vi "Configure Pins.vi"(8 "error in":errorcluster, 11 "2727 in":refnum<class "2727.lvclass">) -> (0 "error out":errorcluster, 3 "2727 out":refnum<class "2727.lvclass">)   [LabVIEW 2019, in "2727.lvlib" / "2727.lvclass"]
uses:
  Library/2727.lvclass
  C:/Users/Public/Documents/Development/builds/Instruments/PRM.lvlibp/Library/PRM.lvclass
  Library/2727.lvclass/2727.ctl
  <instrlib>/ni272xReferenceVIs/ni272xReferenceVIs.llb/ni272x Connector Identifier.ctl
  builds/Instruments/PRM.lvlibp/Accessors/Read NumChans.vi
  <instrlib>/ni272xReferenceVIs/ni272xReferenceVIs.llb/ni272x Connect to Connector 1Chan.vi
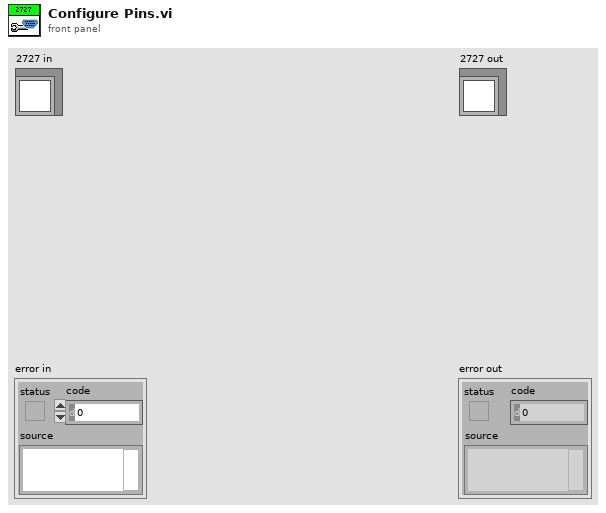
[diagram p1: front panel]
types:
  T1 = typedef "ni272x Connector Identifier.ctl" = enum8{"DUT Connector", "DMM Test Connector"}
  T2 = typedef "ni272x Reference.ctl" = refnum<k20>
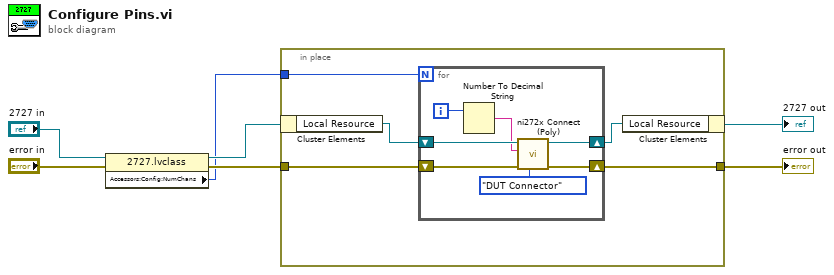
[diagram p0: block diagram]
diagram:
  n1 = property class="2727.lvclass"(reference="2727 in", error in="error in") -> (reference out=w6:refnum<class "2727.lvclass">, error out=w5:errorcluster, "Accessors:Config:NumChans"=w4:i32)
  n2 = in-place {
    in-place-border: w5 -> [w11]
    in-place-border: w4 -> [w10]
    in-place-border: [w8] -> w1
    n3 = in-place-cluster #1(w6) -> ("Local Resource"=w12:T2)
    n4 = for {
      N: w10 -> [_]
      shift-right: [w17] -> w9
      shift-left: w12 -> [w18]
      shift-right: [w15] -> w8
      shift-left: w11 -> [w16]
      i -> [w14]
      n5 = Number To Decimal String(number=w14) -> (decimal integer string=w13:string)  [unwired: 1 in]
      n6 = call-poly <instrlib>:"ni272x Connect (Poly).vi"("connector identifier"=ni272x_Connector_Identifier."DUT Connector", "error in (no error)"=w16, "resistor channel"=w13, "instrument handle"=w18) -> ("error out"=w15:errorcluster, "instrument handle out"=w17:T2)  [unwired: 6 out]
    }
    n7 = in-place-cluster #1("Local Resource"=w9) -> (→"2727 out":refnum<class "2727.lvclass">)
  }
  "error out" <- w1
